vi "EdgeDetection.vi"(6 "Previous Value":i16, 8 "Threshold":dbl, 9 "Analog Input":dbl) -> (0 "Digitized":i16, 2 "Falling Edge":bool, 3 "Rising Edge":bool)   [LabVIEW 2022 SP3]
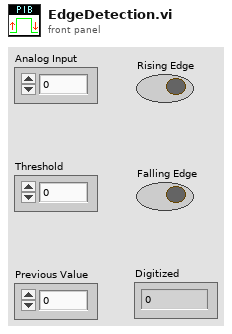
[diagram p1: front panel]
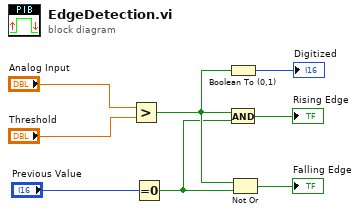
[diagram p0: block diagram]
diagram:
  n1 = Greater?(x="Analog Input", y="Threshold") -> (0:w4:bool)
  n2 = Equal To 0?(x="Previous Value") -> (x = 0?=w1:bool)
  n3 = Boolean To (0,1)(Boolean=w4) -> (0, 1=→"Digitized":i16)
  n4 = And(x=w4, y=w1) -> (x .and. y?=→"Rising Edge":bool)
  n5 = Not Or(1:w1, 2:w4) -> (0:→"Falling Edge":bool)
